vi "GetMotorInput.vi"(7 "Mode":T1, 8 "Slowdown":dbl format="%#_13g", 9 "Brake":dbl format="%#_13g", 10 "Setpoint":dbl format="%#_13g", 11 "Current":dbl format="%#_13g") -> (1 "MotorInput":dbl)   [LabVIEW 2013]
doc: "Determines the needed motor input to get the robot to reach the setpoint. The algorithm is chosen by the mode.\nInputs:\n-Mode: fullspeed or linear scaling\n-Current: the current sensor value\n-Setpoint: the desired value\n-Brake: \"close enough\", i.e. the distance away from the setpoint at which the robot brakes.\n-Slowdown: the distance away from the setpoint that the robot begins to slow down."
uses:
  AutoAlignState.ctl
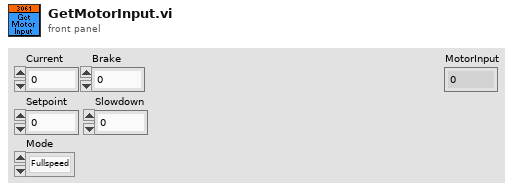
[diagram p1: front panel]
types:
  T1 = typedef "AutoAlignState.ctl" = enum16{"Fullspeed", "Linear"}
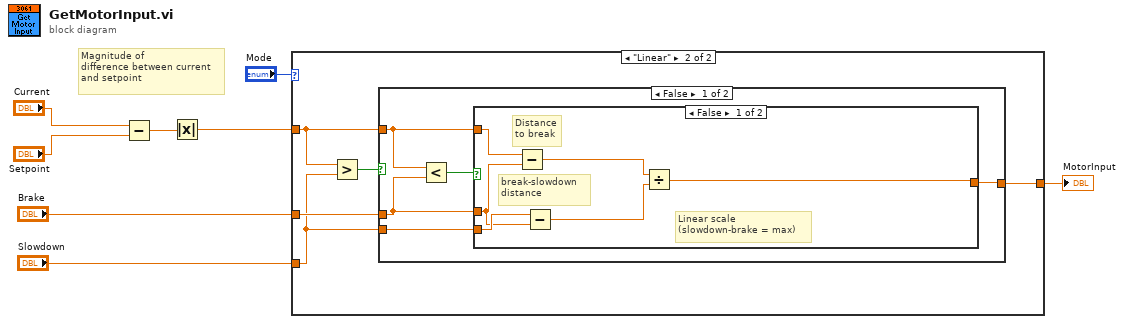
[diagram p0: block diagram]
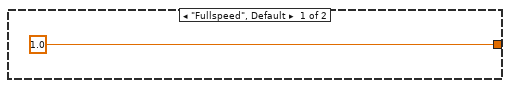
[diagram p2: hidden frame]
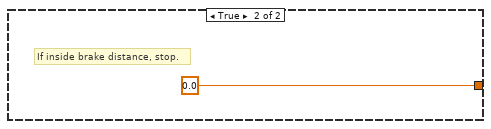
[diagram p3: hidden frame]
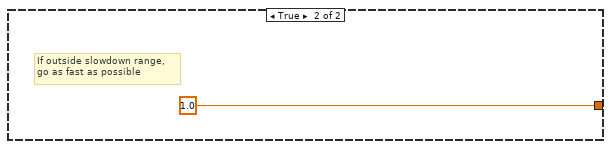
[diagram p4: hidden frame]
diagram:
  # "Magnitude of\ndifference between current\nand setpoint"
  n1 = Subtract(x="Current", y="Setpoint") -> (x-y=w6:dbl)
  n2 = Absolute Value(x=w6) -> (abs(x)=w4:dbl)
  n3 = case shown="\"Linear\"" "Mode" {
    tunnel: w4 -> [_ w11]
    tunnel: "Brake" -> [_ w12]
    tunnel: "Slowdown" -> [_ w10]
    tunnel: [1.0 w13] -> w1
    frame "Fullspeed", Default {
    }
    frame "Linear" {
      n4 = Greater?(x=w11, y=w10) -> (0:w14:bool)
      n5 = case shown="False" w14 {
        tunnel: [w18 1.0] -> w13
        tunnel: w12 -> [w16 _]
        tunnel: w11 -> [w17 _]
        tunnel: w10 -> [w15 _]
        frame False {
          n6 = Less?(x=w17, y=w16) -> (x < y?=w19:bool)
          n7 = case shown="False" w19 {
            tunnel: [w20 0.0] -> w18
            tunnel: w17 -> [w25 _]
            tunnel: w16 -> [w23 _]
            tunnel: w15 -> [w24 _]
            frame False {
              # "Linear scale\n(slowdown-brake = max)"
              # "break-slowdown\ndistance"
              # "Distance\nto break"
              n8 = Subtract(x=w25, y=w23) -> (x-y=w22:dbl)
              n9 = Subtract(x=w24, y=w23) -> (x-y=w21:dbl)
              n10 = Divide(x=w22, y=w21) -> (x/y=w20:dbl)
            }
            frame True {
              # "If inside brake distance, stop."
            }
          }
        }
        frame True {
          # "If outside slowdown range,\ngo as fast as possible"
        }
      }
    }
  }
  "MotorInput" <- w1
